vi "convert_string_to_int32.vi"(3 "default (0)":i32, 4 "String in":string) -> (1 "int32 value out":i32)   [LabVIEW 2014, in "rszvl_rsidr_core.lvlib"]
uses:
  rszvl_rsidr_core.lvlib
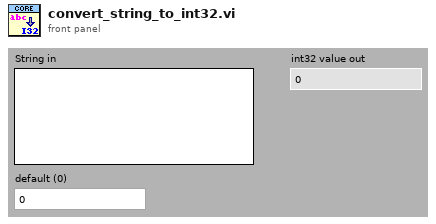
[diagram p1: front panel]
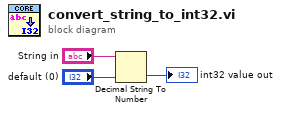
[diagram p0: block diagram]
diagram:
  n1 = Decimal String To Number(string="String in", default (0L)="default (0)") -> (number=→"int32 value out":i32)  [unwired: 1 in, 1 out]
